vi "RunTest.vi"(8 "error in":errorcluster, 11 "Prueba31 in":refnum<class "Prueba33.lvclass">) -> (0 "error out":errorcluster, 2 "Resultado":string, 3 "Prueba31 out":refnum<class "Prueba33.lvclass">)   [LabVIEW 2019, in "Prueba33.lvclass"]
uses:
  Prueba33.lvclass
  Prueba04/Control/Slide.ctl
  Controles/Tab.ctl
  <vilib>/Utility/miscctls.llb/LVRowAndColumnTypeDef.ctl
  Prueba33.lvclass/Prueba33.ctl
  QMH/Message Queue/Enqueue Message (Single).vi
  <vilib>/Utility/error.llb/Error Cluster From Error Code.vi
  <vilib>/ErrorRing/Error Ring.xnode
  QMH/Message Queue/Message Queue.lvlib
  QMH/User Event - Stop/User Event - Stop.lvlib
  Prueba04/Prueba04.lvclass
panel:
  in  "Tab":T1
  out "Estatus_MainD4":string
  in  "Configurar_MainD4":bool
  in  "Ver_MainD4":bool
  out "Estatus_MainD3":string
  in  "Configurar_MainD3":bool
  in  "Ver_MainD3":bool
  out "Estatus_MainD2":string
  in  "Configurar_MainD2":bool
  in  "Ver_MainD2":bool
  out "Estatus_MainD1":string
  in  "Configurar_MainD1":bool
  in  "Ver_MainD1":bool
  in  "Salir_Main":bool
  in  "frecuencia_D1A":string(combo)="63"
  out "NivelendB_D1A":dbl=95.0
  out "rangoRef_D1A":string
  in  "guardarVref_D1A":bool
  in  "generar_D1A":bool
  in  "AjusteAmp_D1A":T2 caption="Ajuste de amplitud [mV]" scale=0.0..5000.0
  out "voltajeM_D1A":dbl format="%#.1f"
  out "frecuenciaM_D1A":dbl format="%#.1f"
  in  "seguir_D1A":bool
  in  "Terminar_D1B":bool
  out "Voltaje_D1B":dbl
  in  "generar_D1B":bool
  out "voltajeM_D1B":dbl format="%#.1f"
  out "frecuenciaM_D1B":dbl format="%#.1f"
  in  "salir_D1B":bool
  in  "Tabla_D1B":string[][](table)=[["63"], ["125"], ["250"], ["500"], ["1000"], ["2000"], ["4000"], ["8000"]]
  in  "frecuencia_D1B":string(combo)="63"
  in  "frecuencia_D2A":string(combo)="63"
  in  "seguir_D2A":bool
  out "voltajeM_D2A":dbl format="%#.1f"
  out "frecuenciaM_D2A":dbl format="%#.1f"
  in  "AjusteAmp_D2A":T2 caption="Ajuste de amplitud [mV]" scale=0.0..5000.0
  in  "generar_D2A":bool
  in  "guardarVref_D2A":bool
  out "rangoRef_D2A":string
  out "NivelendB_D2A":dbl=95.0
  in  "Terminar_D2B":bool
  in  "frecuencia_D2B":string(combo)="63"
  in  "salir_D2B":bool
  out "voltajeM_D2B":dbl format="%#.1f"
  out "frecuenciaM_D2B":dbl format="%#.1f"
  in  "generar_D2B":bool
  out "Voltaje_D2B":dbl
  in  "Tabla_D2B":string[][](table)=[["63"], ["125"], ["250"], ["500"], ["1000"], ["2000"], ["4000"], ["8000"]]
  in  "frecuencia_D3A":string(combo)="63"
  out "NivelendB_D3A":dbl=95.0
  out "rangoRef_D3A":string
  in  "guardarVref_D3A":bool
  in  "generar_D3A":bool
  in  "AjusteAmp_D3A":T2 caption="Ajuste de amplitud [mV]" scale=0.0..5000.0
  out "voltajeM_D3A":dbl format="%#.1f"
  out "frecuenciaM_D3A":dbl format="%#.1f"
  in  "seguir_D3A":bool
  in  "Terminar_D3B":bool
  in  "frecuencia_D3B":string(combo)="63"
  in  "Tabla_D3B":string[][](table)=[["63"], ["125"], ["250"], ["500"], ["1000"], ["2000"], ["4000"], ["8000"]]
  out "Voltaje_D3B":dbl
  in  "generar_D3B":bool
  out "voltajeM_D3B":dbl format="%#.1f"
  out "frecuenciaM_D3B":dbl format="%#.1f"
  in  "salir_D3B":bool
  in  "frecuencia_D4A":string(combo)="63"
  in  "seguir_D4A":bool
  out "voltajeM_D4A":dbl format="%#.1f"
  out "frecuenciaM_D4A":dbl format="%#.1f"
  in  "AjusteAmp_D4A":T2 caption="Ajuste de amplitud [mV]" scale=0.0..5000.0
  in  "generar_D4A":bool
  in  "guardarVref_D4A":bool
  out "rangoRef_D4A":string
  out "NivelendB_D4A":dbl=95.0
  in  "Terminar_D4B":bool
  in  "salir_D4B":bool
  out "voltajeM_D4B":dbl format="%#.1f"
  out "frecuenciaM_D4B":dbl format="%#.1f"
  in  "generar_D4B":bool
  out "Voltaje_D4B":dbl
  in  "Tabla_D4B":string[][](table)=[["63"], ["125"], ["250"], ["500"], ["1000"], ["2000"], ["4000"], ["8000"]]
  in  "frecuencia_D4B":string(combo)="63"
  # "Vienen de base de datos\nambos\ncambiar a numerico indicador"
  # "Dosimetro 4"
  # "Dosimetro 3"
  # "Dosimetro 2"
  # "Dosimetro 1"
  # "3.  Ponderación frecuencial A (entrada eléctrica). . IEC 61252: 2002 Cláusula 7"
  # "Elección Señal de Referencia\nsegún marca y modelo de sonómetro"
  # "Nivel en dB"
  # "Rango Referencia"
  # "Frecuencia"
  # "Monitoreo"
  # "Frecuencia"
  # "Hz"
  # "Voltaje"
  # "mV"
  # "3.  Ponderación frecuencial A (entrada eléctrica). . IEC 61252: 2002 Cláusula 7\nDosimetro 1"
  # "Tabla Resultados"
  # "3.  Ponderación frecuencial A (entrada eléctrica). . IEC 61252: 2002 Cláusula 7\nDosimetro 1"
  # "Voltaje"
  # "Frecuencia"
  # "Monitoreo"
  # "Frecuencia"
  # "Hz"
  # "Voltaje"
  # "mV"
  # "Elección Señal de Referencia\nsegún marca y modelo de sonómetro"
  # "3.  Ponderación frecuencial A (entrada eléctrica). . IEC 61252: 2002 Cláusula 7\nDosimetro 2"
  # "Monitoreo"
  # "Frecuencia"
  # "Hz"
  # "Voltaje"
  # "mV"
  # "Frecuencia"
  # "Rango Referencia"
  # "Nivel en dB"
  # "Tabla Resultados"
  # "3.  Ponderación frecuencial A (entrada eléctrica). . IEC 61252: 2002 Cláusula 7\nDosimetro 2"
  # "Monitoreo"
  # "Frecuencia"
  # "Hz"
  # "Voltaje"
  # "mV"
  # "Frecuencia"
  # "Voltaje"
  # "Elección Señal de Referencia\nsegún marca y modelo de sonómetro"
  # "3.  Ponderación frecuencial A (entrada eléctrica). . IEC 61252: 2002 Cláusula 7\nDosimetro 3"
  # "Nivel en dB"
  # "Rango Referencia"
  # "Frecuencia"
  # "Monitoreo"
  # "Frecuencia"
  # "Hz"
  # "Voltaje"
  # "mV"
  # "Tabla Resultados"
  # "3.  Ponderación frecuencial A (entrada eléctrica). . IEC 61252: 2002 Cláusula 7\nDosimetro 3"
  # "Voltaje"
  # "Frecuencia"
  # "Monitoreo"
  # "Frecuencia"
  # "Hz"
  # "Voltaje"
  # "mV"
  # "Elección Señal de Referencia\nsegún marca y modelo de sonómetro"
  # "3.  Ponderación frecuencial A (entrada eléctrica). . IEC 61252: 2002 Cláusula 7\nDosimetro 4"
  # "Monitoreo"
  # "Frecuencia"
  # "Hz"
  # "Voltaje"
  # "mV"
  # "Frecuencia"
  # "Rango Referencia"
  # "Nivel en dB"
  # "Tabla Resultados"
  # "Monitoreo"
  # "Frecuencia"
  # "Hz"
  # "Voltaje"
  # "mV"
  # "Frecuencia"
  # "Voltaje"
  # "3.  Ponderación frecuencial A (entrada eléctrica). . IEC 61252: 2002 Cláusula 7\nDosimetro 4"
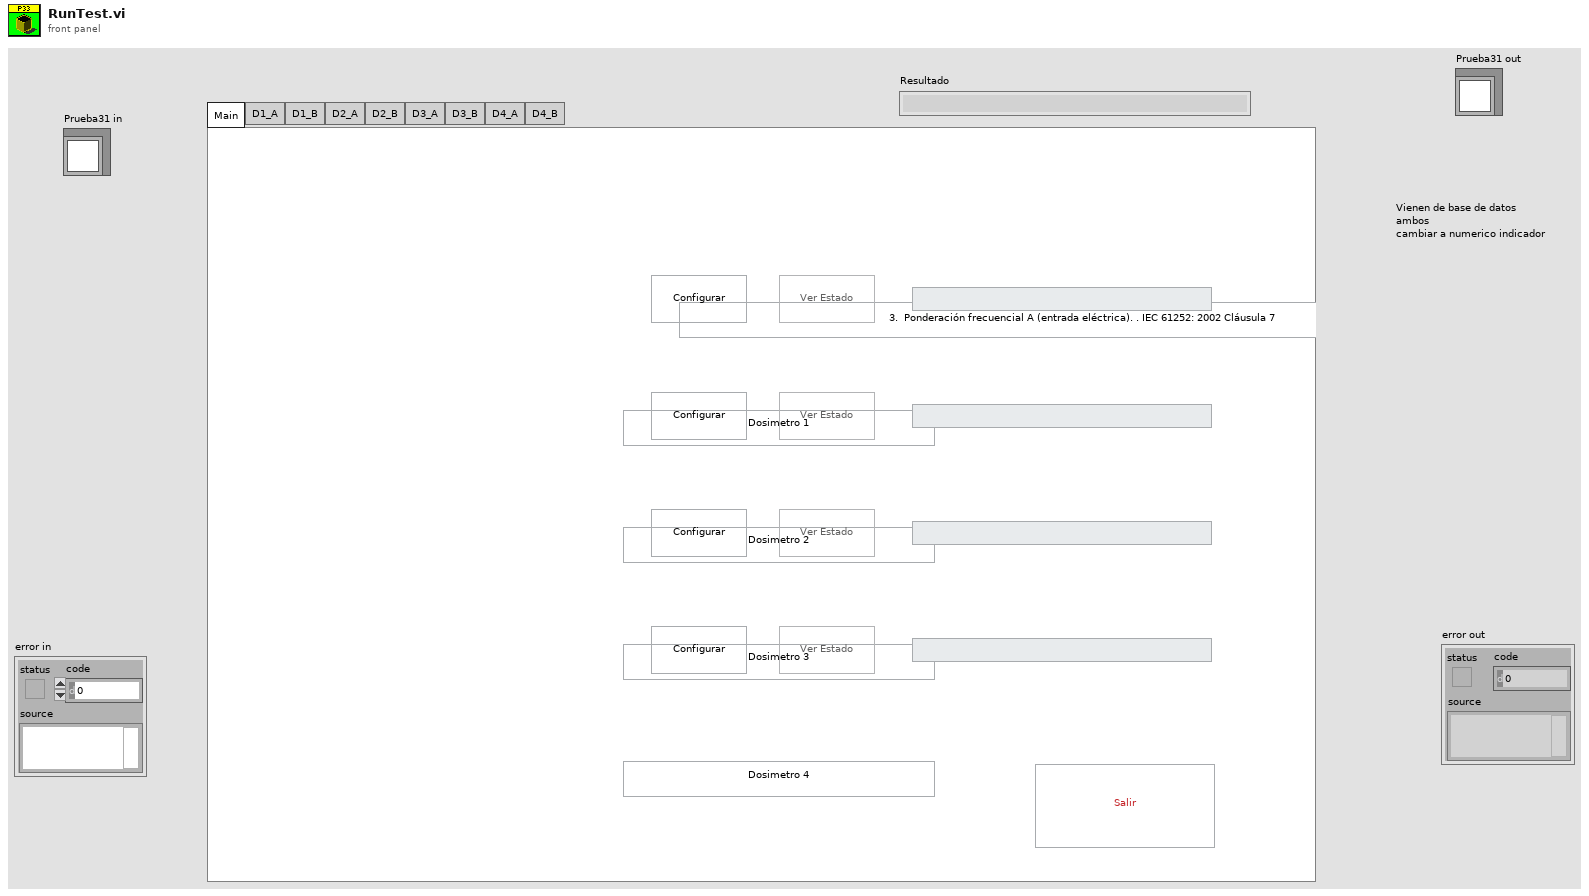
[diagram p1: front panel]
types:
  T1 = typedef "Prueba33.lvclass/Tab.ctl" = enum32{"Main", "D1_A", "D1_B", "D2_A", "D2_B", "D3_A", "D3_B", "D4_A", "D4_B"}
  T2 = typedef "Prueba04.lvclass/Slide.ctl" = dbl
  T3 = typedef "Message Queue.lvlib/All Message Queues.ctl" = cluster{"MHL":refnum<queue>, "Inst_CNT90":refnum<queue>, "Inst_DS360":refnum<queue>, "Inst_Keithley2002":refnum<queue>, "Inst_DAQ":refnum<queue>, "BD":refnum<queue>, "Pistofono":refnum<queue>, "Nexus":refnum<queue>}
  T4 = typedef "LVRowAndColumnTypeDef.ctl" = cluster{"Row":i32, "Column":i32}
  T5 = cluster{"Channel 1":cluster{"amplitude":dbl, "detected fundamental frequency":dbl}, "Channel 2":cluster{"amplitude":dbl, "detected fundamental frequency":dbl}, "Channel 3":cluster{"amplitude":dbl, "detected fundamental frequency":dbl}, "Channel 4":cluster{"amplitude":dbl, "detected fundamental frequency":dbl}}
  T6 = cluster{"Vref":dbl, "Frecuencia":dbl, "Channel":string}
  T7 = cluster{"Vref_D1":dbl, "Vref_D2":dbl, "Vref_D3":dbl, "Vref_D4":dbl}
  T8 = cluster{"ControlName":string, "ControlReference":refnum<vi>}[]
  T9 = enum16{"Tabla_D1", "Tabla_D2", "Tabla_D3", "Tabla_D4"}[]
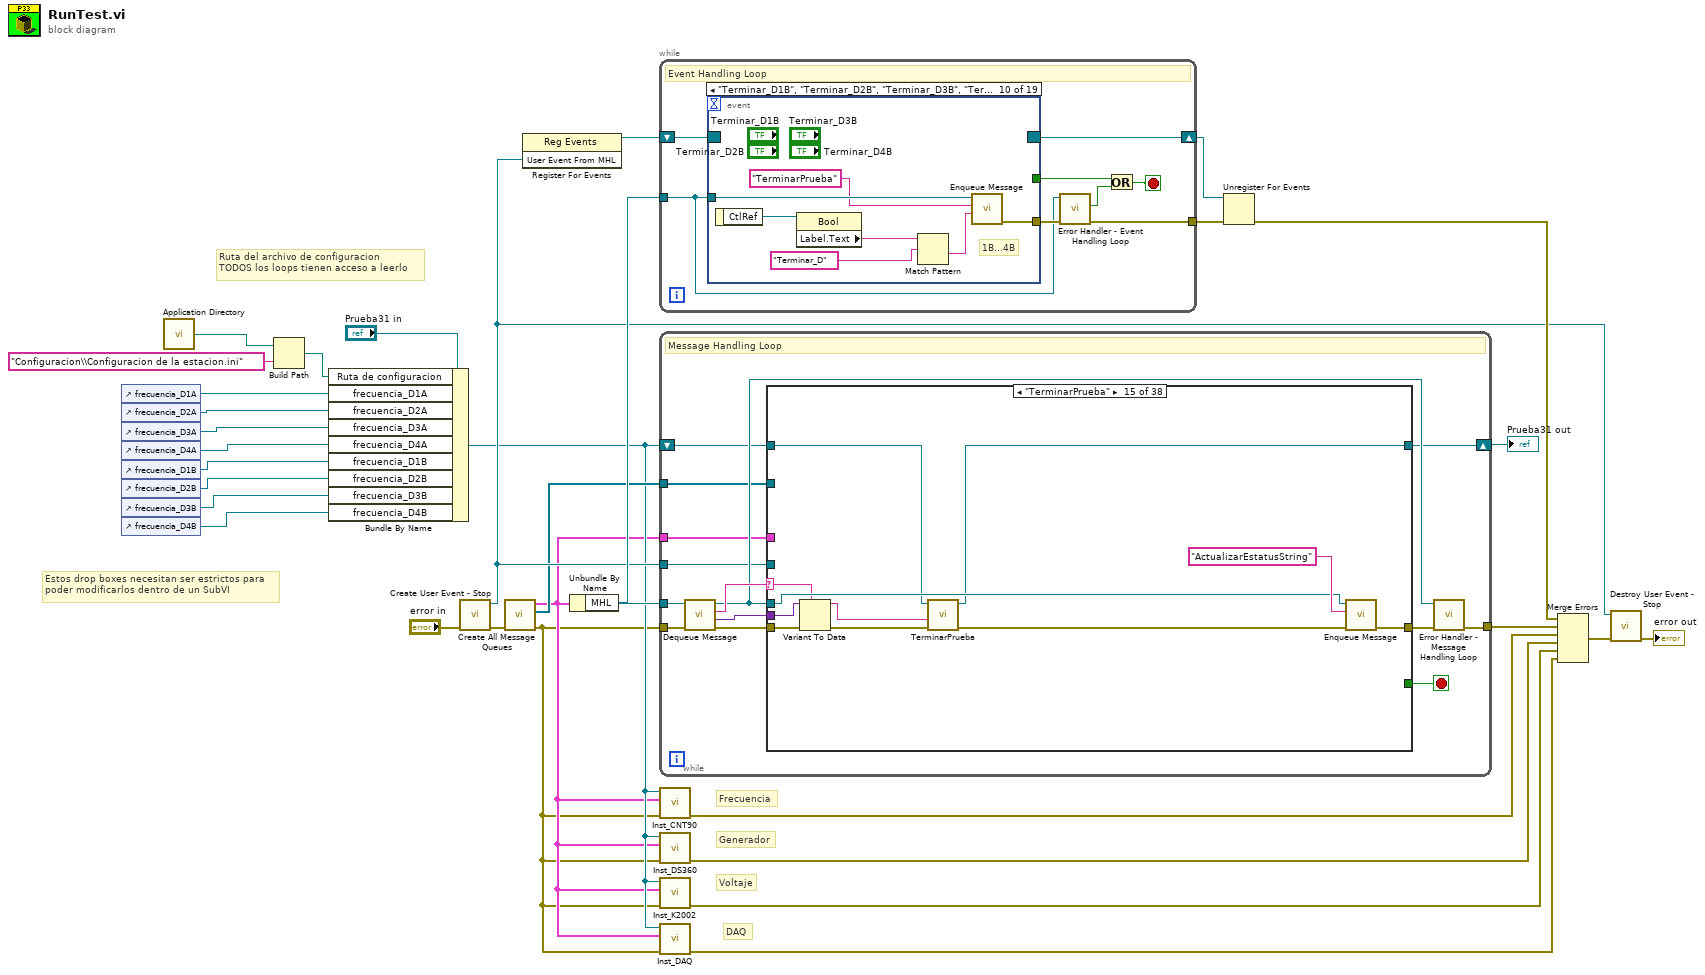
[diagram p0: block diagram]
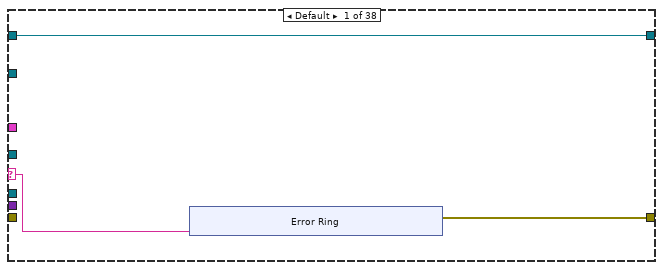
[diagram p2: hidden frame]
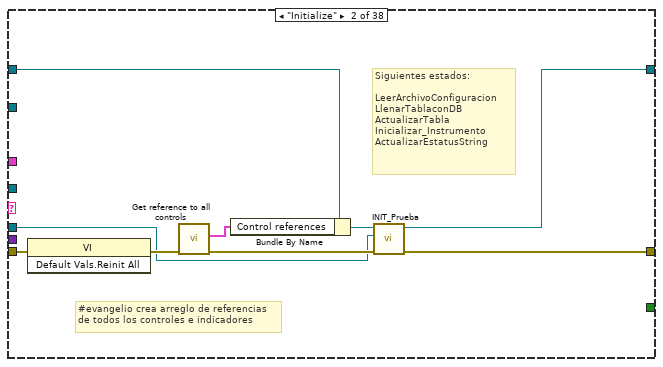
[diagram p3: hidden frame]
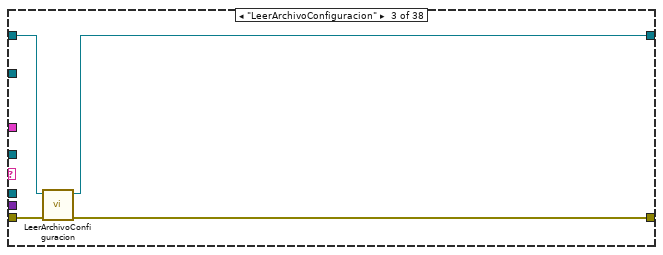
[diagram p4: hidden frame]
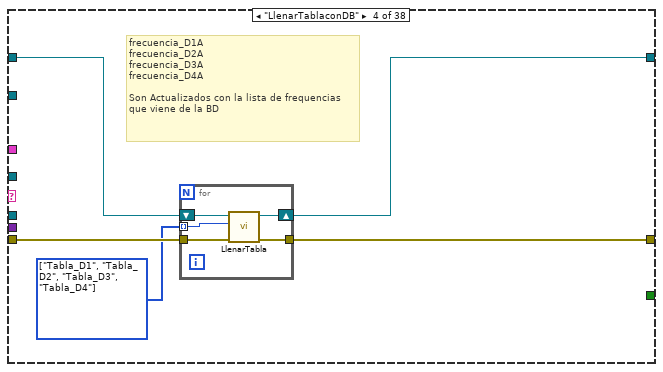
[diagram p5: hidden frame]
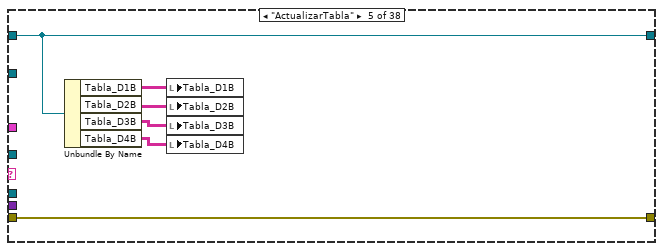
[diagram p6: hidden frame]
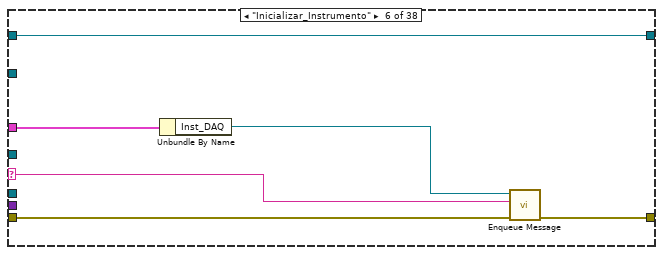
[diagram p7: hidden frame]
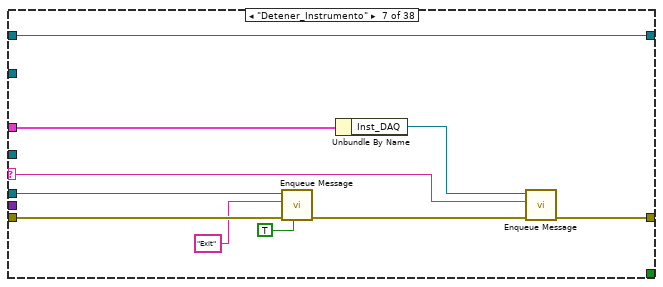
[diagram p8: hidden frame]
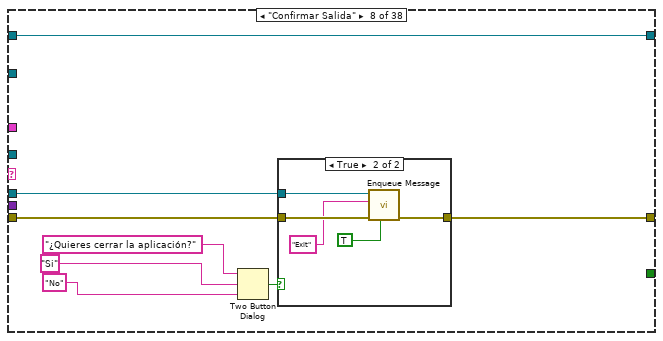
[diagram p9: hidden frame]
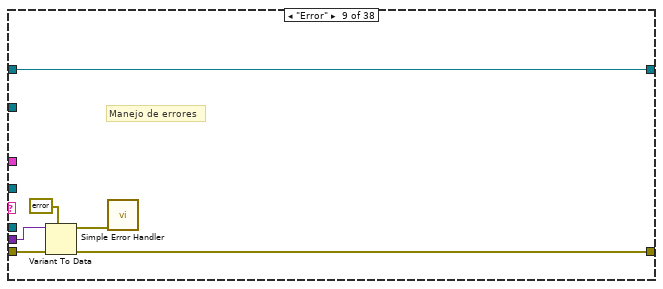
[diagram p11: hidden frame]
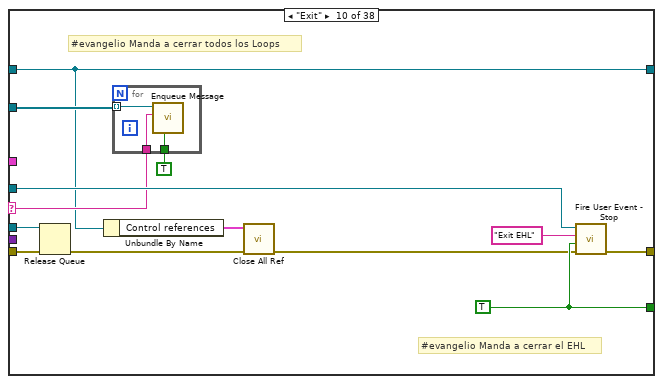
[diagram p12: hidden frame]
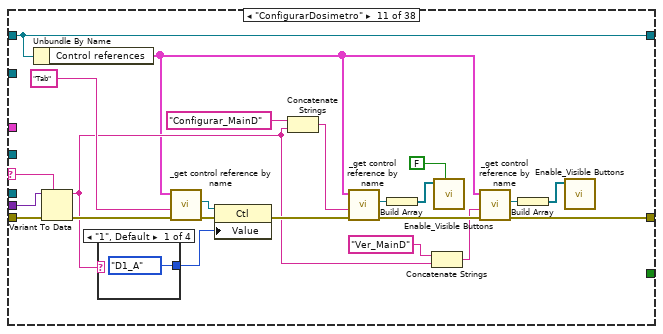
[diagram p13: hidden frame]
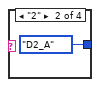
[diagram p14: hidden frame]
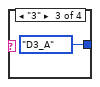
[diagram p15: hidden frame]
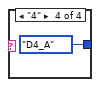
[diagram p16: hidden frame]
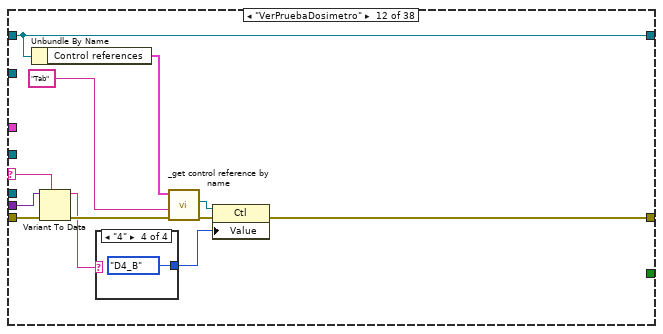
[diagram p17: hidden frame]
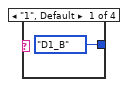
[diagram p18: hidden frame]
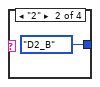
[diagram p19: hidden frame]
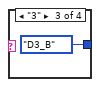
[diagram p20: hidden frame]
diagram:
  # "Ruta del archivo de configuracion\nTODOS los loops tienen acceso a leerlo"
  # "Estos drop boxes necesitan ser estrictos para\npoder modificarlos dentro de un SubVI"
  # "DAQ"
  # "Generador"
  # "Voltaje"
  # "Frecuencia"
  n1 = control-ref of="frecuencia_D1A"() -> (w8:refnum<vi>)
  n2 = control-ref of="frecuencia_D2A"() -> (w7:refnum<vi>)
  n3 = control-ref of="frecuencia_D3A"() -> (w6:refnum<vi>)
  n4 = control-ref of="frecuencia_D4A"() -> (w5:refnum<vi>)
  n5 = control-ref of="frecuencia_D1B"() -> (w4:refnum<vi>)
  n6 = control-ref of="frecuencia_D2B"() -> (w3:refnum<vi>)
  n7 = control-ref of="frecuencia_D3B"() -> (w2:refnum<vi>)
  n8 = control-ref of="frecuencia_D4B"() -> (w1:refnum<vi>)
  n9 = call <vilib>:"Application Directory.vi"() -> ("Application Directory"=w16:path)
  n10 = Build Path(base path=w16, name or relative path="Configuracion\\Configuracion de la estacion.ini") -> (appended path=w15:path)
  n11 = Bundle By Name(cluster="Prueba31 in", "Ruta de configuracion"=w15, "frecuencia_D1A"=w8, "frecuencia_D2A"=w7, "frecuencia_D3A"=w6, "frecuencia_D4A"=w5, "frecuencia_D1B"=w4, "frecuencia_D2B"=w3, "frecuencia_D3B"=w2, "frecuencia_D4B"=w1) -> (w12:refnum<class "Prueba33.lvclass">)
  n12 = call "Create User Event - Stop.vi"("error in (no error)"="error in") -> ("error out"=w29:errorcluster, "User Event From MHL"=w23:refnum<user-event>)  [unwired: 9 in]
  n13 = call "Create All Message Queues.vi"("error in (no error)"=w29) -> ("error out"=w10:errorcluster, "PL Queues Array"=w13:refnum<queue>[], "All Message Queues out"=w11:T3)  [unwired: 8 in]
  n14 = register-events(w23) -> (reference out=w32:refnum<event-registration>)  [unwired: 2 in, 1 out]
  n15 = Unbundle By Name(w11) -> ("MHL"=w28:refnum<queue>)
  n16 = while {
    tunnel: w28 -> [w33]
    tunnel: [w37] -> w31
    shift-right: [w39] -> w30
    shift-left: w32 -> [w40]
    stop <- w34 stop-if-true
    # "Event Handling Loop"
    n17 = event shown="[9] \"Terminar_D1B\", \"Terminar_D2B\", \"Terminar_D3B\", \"Terminar_D4B\": Value Change" {
      selector: w40 -> [_ _ _ _ _ _ _ _ _ _ _ _ _ _ _ _ _ _ _]
      dyn-events: [_ _ _ _ _ _ _ _ _ _ _ _ _ _ _ _ _ _ _] -> w39
      timeout: _ -> [_ _ _ _ _ _ _ _ _ _ _ _ _ _ _ _ _ _ _]
      tunnel: w33 -> [w43 _ w52 w59 w66 w73 w80 w87 w94 w101 w110 w121 w131 w141 w151 w161 w171 w181 w183]
      tunnel: [w44 _ w53 w60 w67 w74 w81 w88 w95 w102 w111 w122 w132 w142 w152 w162 w172 w182 w192] -> w38
      tunnel: [_ w45 _ _ _ _ _ _ _ _ _ _ _ _ _ _ _ _ _] -> w35
      event Panel Close? {
        w41 = TRUE
        n18 = event-data() -> ()  [unwired: 1 in, 1 out]
        n19 = call-poly "Enqueue Message.vi"("Priority Message? (F)"=w41, "Message"="Confirmar Salida", "Message Queue"=w43) -> ("error out"=w44:errorcluster)  [unwired: 7 in, 1 out]
        n20 = event-data("Discard?"=w41) -> ()  [unwired: 1 in, 1 out]
      }
      event User Event {
        n21 = event-data() -> ("User Event"=w47:string, "Event Data"=w46:variant)  [unwired: 1 in]
        n22 = case shown="Default" w47 {
          tunnel: w46 -> [_ w49]
          tunnel: [_ w48] -> w45
          frame Default {
          }
          frame "Exit EHL" {
            # "#evangelio Termina\nla ejecucion del EHL"
            n23 = Variant To Data(type=TRUE, Variant=w49) -> (data=w48:bool)  [unwired: 1 in, 1 out]
          }
        }
      }
      event "Salir_Main": Value Change {
        n24 = event-data() -> ()  [unwired: 1 in, 1 out]
        n25 = call-poly "Enqueue Message.vi"("Message"="Detener_Instrumento", "Message Queue"=w52) -> ("error out"=w53:errorcluster)  [unwired: 8 in, 1 out]
      }
      event "Configurar_MainD1", "Configurar_MainD2", "Configurar_MainD3", "Configurar_MainD4": Value Change {
        n26 = event-data() -> ("CtlRef"=w57:refnum<vi>)  [unwired: 1 in]
        n27 = property class="Bool"(reference=w57) -> ("Label.Text"=w56:string)  [unwired: 1 in, 2 out]
        n28 = Match Pattern(string=w56, regular expression="Configurar_MainD" ("Message")) -> (after substring=w54:string)  [unwired: 1 in, 3 out]
        n29 = call-poly "Enqueue Message.vi"("Message Data"=w54, "Message"="ConfigurarDosimetro", "Message Queue"=w59) -> ("error out"=w60:errorcluster)  [unwired: 7 in, 1 out]
      }
      event "Ver_MainD1", "Ver_MainD2", "Ver_MainD3", "Ver_MainD4": Value Change {
        n30 = event-data() -> ("CtlRef"=w64:refnum<vi>)  [unwired: 1 in]
        n31 = property class="Bool"(reference=w64) -> ("Label.Text"=w63:string)  [unwired: 1 in, 2 out]
        n32 = Match Pattern(string=w63, regular expression="Ver_MainD" ("Message")) -> (after substring=w61:string)  [unwired: 1 in, 3 out]
        n33 = call-poly "Enqueue Message.vi"("Message Data"=w61, "Message"="VerPruebaDosimetro", "Message Queue"=w66) -> ("error out"=w67:errorcluster)  [unwired: 7 in, 1 out]
      }
      event "seguir_D1A", "seguir_D2A", "seguir_D3A", "seguir_D4A": Value Change {
        n34 = event-data() -> ("CtlRef"=w71:refnum<vi>)  [unwired: 1 in]
        n35 = property class="Bool"(reference=w71) -> ("Label.Text"=w70:string)  [unwired: 1 in, 2 out]
        n36 = Match Pattern(string=w70, regular expression="seguir_D" ("Message")) -> (after substring=w68:string)  [unwired: 1 in, 3 out]
        n37 = call-poly "Enqueue Message.vi"("Message Data"=w68, "Message"="MoveraPruebaB", "Message Queue"=w73) -> ("error out"=w74:errorcluster)  [unwired: 7 in, 1 out]
      }
      event "salir_D1B", "salir_D2B", "salir_D3B", "salir_D4B": Value Change {
        n38 = event-data() -> ("CtlRef"=w78:refnum<vi>)  [unwired: 1 in]
        n39 = property class="Bool"(reference=w78) -> ("Label.Text"=w77:string)  [unwired: 1 in, 2 out]
        n40 = Match Pattern(string=w77, regular expression="salir_D" ("Message")) -> (after substring=w75:string)  [unwired: 1 in, 3 out]
        n41 = call-poly "Enqueue Message.vi"("Message Data"=w75, "Message"="MoveraPruebaMain", "Message Queue"=w80) -> ("error out"=w81:errorcluster)  [unwired: 7 in, 1 out]
      }
      event Value Change {
        # "1A...4A"
        n42 = event-data() -> ("CtlRef"=w85:refnum<vi>)  [unwired: 1 in]
        n43 = property class="Slide (strict)"(reference=w85) -> ("Label.Text"=w84:string)  [unwired: 1 in, 2 out]
        n44 = Match Pattern(string=w84, regular expression="AjusteAmp_D" ("Message")) -> (after substring=w82:string)  [unwired: 1 in, 3 out]
        n45 = call-poly "Enqueue Message.vi"("Message Data"=w82, "Message"="AjustarAmplitud", "Message Queue"=w87) -> ("error out"=w88:errorcluster)  [unwired: 7 in, 1 out]
      }
      event "guardarVref_D1A", "guardarVref_D2A", "guardarVref_D3A", "guardarVref_D4A": Value Change {
        # "1A...4A"
        n46 = event-data() -> ("CtlRef"=w92:refnum<vi>)  [unwired: 1 in]
        n47 = property class="Bool"(reference=w92) -> ("Label.Text"=w91:string)  [unwired: 1 in, 2 out]
        n48 = Match Pattern(string=w91, regular expression="guardarVref_D" ("Message")) -> (after substring=w89:string)  [unwired: 1 in, 3 out]
        n49 = call-poly "Enqueue Message.vi"("Message Data"=w89, "Message"="GuardarVref", "Message Queue"=w94) -> ("error out"=w95:errorcluster)  [unwired: 7 in, 1 out]
      }
      event "Terminar_D1B", "Terminar_D2B", "Terminar_D3B", "Terminar_D4B": Value Change {
        # "1B...4B"
        n50 = event-data() -> ("CtlRef"=w99:refnum<vi>)  [unwired: 1 in]
        n51 = property class="Bool"(reference=w99) -> ("Label.Text"=w98:string)  [unwired: 1 in, 2 out]
        n52 = Match Pattern(string=w98, regular expression="Terminar_D" ("Message")) -> (after substring=w96:string)  [unwired: 1 in, 3 out]
        n53 = call-poly "Enqueue Message.vi"("Message Data"=w96, "Message"="TerminarPrueba", "Message Queue"=w101) -> ("error out"=w102:errorcluster)  [unwired: 7 in, 1 out]
      }
      event "generar_D1A": Value Change {
        # "1A...4A"
        n54 = event-data() -> ("CtlRef"=w104:refnum<vi>)  [unwired: 1 in]
        n55 = property class="Bool (strict)"(reference=w104) -> ("Label.Text"=w106:string)  [unwired: 1 in, 2 out]
        n56 = Select(t="SetDAQ_AO", s="generar_D1A", f="DetenerMonitor") -> (s? t:f=w107:string)
        n57 = Match Pattern(string=w106, regular expression="generar_D" ("Message")) -> (after substring=w103:string)  [unwired: 1 in, 3 out]
        n58 = call-poly "Enqueue Message.vi"("Message Data"=w103, "Message"=w107, "Message Queue"=w110) -> ("error out"=w111:errorcluster)  [unwired: 7 in, 1 out]
      }
      event "generar_D2A": Value Change {
        # "1A...4A"
        n59 = event-data() -> ("CtlRef"=w115:refnum<vi>)  [unwired: 1 in]
        n60 = property class="Bool (strict)"(reference=w115) -> ("Label.Text"=w117:string)  [unwired: 1 in, 2 out]
        n61 = Select(t="SetDAQ_AO", s="generar_D2A", f="DetenerMonitor") -> (s? t:f=w118:string)
        n62 = Match Pattern(string=w117, regular expression="generar_D" ("Message")) -> (after substring=w114:string)  [unwired: 1 in, 3 out]
        n63 = call-poly "Enqueue Message.vi"("Message Data"=w114, "Message"=w118, "Message Queue"=w121) -> ("error out"=w122:errorcluster)  [unwired: 7 in, 1 out]
      }
      event "generar_D3A": Value Change {
        # "1A...4A"
        n64 = event-data() -> ("CtlRef"=w125:refnum<vi>)  [unwired: 1 in]
        n65 = property class="Bool (strict)"(reference=w125) -> ("Label.Text"=w127:string)  [unwired: 1 in, 2 out]
        n66 = Select(t="SetDAQ_AO", s="generar_D3A", f="DetenerMonitor") -> (s? t:f=w128:string)
        n67 = Match Pattern(string=w127, regular expression="generar_D" ("Message")) -> (after substring=w124:string)  [unwired: 1 in, 3 out]
        n68 = call-poly "Enqueue Message.vi"("Message Data"=w124, "Message"=w128, "Message Queue"=w131) -> ("error out"=w132:errorcluster)  [unwired: 7 in, 1 out]
      }
      event "generar_D4A": Value Change {
        # "1A...4A"
        n69 = event-data() -> ("CtlRef"=w135:refnum<vi>)  [unwired: 1 in]
        n70 = property class="Bool (strict)"(reference=w135) -> ("Label.Text"=w137:string)  [unwired: 1 in, 2 out]
        n71 = Select(t="SetDAQ_AO", s="generar_D4A", f="DetenerMonitor") -> (s? t:f=w138:string)
        n72 = Match Pattern(string=w137, regular expression="generar_D" ("Message")) -> (after substring=w134:string)  [unwired: 1 in, 3 out]
        n73 = call-poly "Enqueue Message.vi"("Message Data"=w134, "Message"=w138, "Message Queue"=w141) -> ("error out"=w142:errorcluster)  [unwired: 7 in, 1 out]
      }
      event "generar_D1B": Value Change {
        # "1B...4B"
        n74 = event-data() -> ("CtlRef"=w145:refnum<vi>)  [unwired: 1 in]
        n75 = property class="Bool (strict)"(reference=w145) -> ("Label.Text"=w147:string)  [unwired: 1 in, 2 out]
        n76 = Select(t="SetDAQ_AO", s="generar_D1B", f="DetenerMonitor") -> (s? t:f=w148:string)
        n77 = Match Pattern(string=w147, regular expression="generar_D" ("Message")) -> (after substring=w144:string)  [unwired: 1 in, 3 out]
        n78 = call-poly "Enqueue Message.vi"("Message Data"=w144, "Message"=w148, "Message Queue"=w151) -> ("error out"=w152:errorcluster)  [unwired: 7 in, 1 out]
      }
      event "generar_D2B": Value Change {
        # "1B...4B"
        n79 = event-data() -> ("CtlRef"=w155:refnum<vi>)  [unwired: 1 in]
        n80 = property class="Bool (strict)"(reference=w155) -> ("Label.Text"=w157:string)  [unwired: 1 in, 2 out]
        n81 = Select(t="SetDAQ_AO", s="generar_D2B", f="DetenerMonitor") -> (s? t:f=w158:string)
        n82 = Match Pattern(string=w157, regular expression="generar_D" ("Message")) -> (after substring=w154:string)  [unwired: 1 in, 3 out]
        n83 = call-poly "Enqueue Message.vi"("Message Data"=w154, "Message"=w158, "Message Queue"=w161) -> ("error out"=w162:errorcluster)  [unwired: 7 in, 1 out]
      }
      event "generar_D3B": Value Change {
        # "1B...4B"
        n84 = event-data() -> ("CtlRef"=w165:refnum<vi>)  [unwired: 1 in]
        n85 = property class="Bool (strict)"(reference=w165) -> ("Label.Text"=w167:string)  [unwired: 1 in, 2 out]
        n86 = Select(t="SetDAQ_AO", s="generar_D3B", f="DetenerMonitor") -> (s? t:f=w168:string)
        n87 = Match Pattern(string=w167, regular expression="generar_D" ("Message")) -> (after substring=w164:string)  [unwired: 1 in, 3 out]
        n88 = call-poly "Enqueue Message.vi"("Message Data"=w164, "Message"=w168, "Message Queue"=w171) -> ("error out"=w172:errorcluster)  [unwired: 7 in, 1 out]
      }
      event "generar_D4B": Value Change {
        # "1B...4B"
        n89 = event-data() -> ("CtlRef"=w175:refnum<vi>)  [unwired: 1 in]
        n90 = property class="Bool (strict)"(reference=w175) -> ("Label.Text"=w177:string)  [unwired: 1 in, 2 out]
        n91 = Select(t="SetDAQ_AO", s="generar_D4B", f="DetenerMonitor") -> (s? t:f=w178:string)
        n92 = Match Pattern(string=w177, regular expression="generar_D" ("Message")) -> (after substring=w174:string)  [unwired: 1 in, 3 out]
        n93 = call-poly "Enqueue Message.vi"("Message Data"=w174, "Message"=w178, "Message Queue"=w181) -> ("error out"=w182:errorcluster)  [unwired: 7 in, 1 out]
      }
      event "Tabla_D1B", "Tabla_D2B", "Tabla_D3B", "Tabla_D4B": Value Change {
        # "1B...4B"
        n94 = event-data() -> ("CtlRef"=w191:refnum<vi>)  [unwired: 1 in]
        n95 = property class="Tbl (strict)"(reference=w191) -> ("Selection Start"=w186:T4, "Label.Text"=w188:string)  [unwired: 1 in, 2 out]
        n96 = Match Pattern(string=w188, regular expression="Tabla_D" ("Message")) -> (after substring=w185:string)  [unwired: 1 in, 3 out]
        n97 = Bundle By Name(cluster=cluster{"Tabla":string, "Posicion":T4} {"Tabla"="", "Posicion"={"Row"=0, "Column"=0}}, "Posicion"=w186, "Tabla"=w185) -> (w184:cluster{"Tabla":string, "Posicion":T4})
        n98 = call-poly "Enqueue Message.vi"("Message Data"=w184, "Message"="EvaluarTabla", "Message Queue"=w183) -> ("error out"=w192:errorcluster)  [unwired: 7 in, 1 out]
      }
    }
    n99 = call "Error Handler - Event Handling Loop.vi"("error in (no error)"=w38, "Message Queue"=w33) -> ("dup error in"=w37:errorcluster, "Error?"=w36:bool)  [unwired: 7 in, 1 out]
    n100 = Or(x=w35, y=w36) -> (x .or. y?=w34:bool)
  }
  n101 = while {
    tunnel: w10 -> [w206]
    tunnel: w28 -> [w205]
    tunnel: [w199] -> w26
    shift-right: [w197] -> w24
    shift-left: w12 -> [w198]
    tunnel: w11 -> [w195]
    tunnel: w23 -> [w194]
    tunnel: w13 -> [w193]
    stop <- w196 stop-if-true
    # "Message Handling Loop"
    n102 = call "Dequeue Message.vi"("error in (no error)"=w206, "Message Queue"=w205) -> ("error out"=w202:errorcluster, "Message Data"=w203:variant, "Message"=w204:string, "dup Message Queue"=w201:refnum<queue>)  [unwired: 6 in]
    n103 = case shown="\"TerminarPrueba\"" w204 {
      selector: w204 -> [w208 _ _ _ _ w246 w257 _ _ w286 w318 w326 w346 w371 w394 _ _ _ _ _ _ _ w452 w486 w512 w546 _ _ _ _ _ _ _ _ _ _ _ _]
      tunnel: w201 -> [_ w218 _ _ _ _ w254 w262 _ w293 _ _ _ w367 w397 _ _ _ _ _ _ _ _ _ _ _ _ _ _ _ _ _ _ _ _ _ _ _]
      tunnel: w203 -> [_ _ _ _ _ _ _ _ w277 _ w319 w327 w347 w372 w393 _ _ w420 _ _ _ w442 w460 w489 w517 w550 w560 _ _ _ _ _ _ _ _ _ _ _]
      tunnel: w202 -> [_ w225 w229 w234 w245 w249 w255 w268 w278 w292 w320 w328 w348 w373 w395 w407 w413 w421 w423 w427 w433 w443 w459 w490 w518 w551 w561 w564 w566 w568 w570 w572 w574 w576 w578 w580 w582 w584]
      tunnel: [w207 w217 w226 w231 w245 w250 w260 w267 w279 w290 w300 w325 w344 w368 w398 w407 w413 w417 w423 w428 w434 w439 w455 w494 w513 w547 w562 w564 w566 w568 w570 w572 w574 w576 w578 w580 w582 w584] -> w200
      tunnel: w198 -> [w209 w223 w228 w233 w244 w251 w261 w269 w281 w283 w317 w329 w349 w364 w392 w405 w412 w416 w422 w429 w435 w436 w451 w485 w508 w539 w556 w563 w565 w567 w569 w571 w573 w575 w577 w579 w581 w583]
      tunnel: [w209 w220 w227 w232 w244 w251 w261 w269 w281 w283 w317 w329 w349 w365 w391 w406 w412 w415 w422 w429 w435 w437 w450 w485 w508 w539 w557 w563 w565 w567 w569 w571 w573 w575 w577 w579 w581 w583] -> w197
      tunnel: [_ _ _ _ _ _ _ _ _ w287 _ _ _ _ _ _ _ _ _ _ _ _ _ _ _ _ _ _ _ _ _ _ _ _ _ _ _ _] -> w196
      tunnel: w195 -> [_ _ _ _ _ w248 w259 _ _ _ _ _ w342 _ _ _ _ _ _ w426 w432 _ w454 w493 w510 w544 _ _ _ _ _ _ _ _ _ _ _ _]
      tunnel: w194 -> [_ _ _ _ _ _ _ _ _ w289 _ _ _ _ _ _ _ _ _ _ _ _ _ _ _ _ _ _ _ _ _ _ _ _ _ _ _ _]
      tunnel: w193 -> [_ _ _ _ _ _ _ _ _ w284 _ _ _ _ _ _ _ _ _ _ _ _ _ _ _ _ _ _ _ _ _ _ _ _ _ _ _ _]
      frame Default {
        n104 = xnode "Error Ring"("parameter 0"=w208) -> ("error out"=w207:errorcluster)
      }
      frame "Initialize" {
        # "Siguientes estados:\n\nLeerArchivoConfiguracion\nLlenarTablaconDB\nActualizarTabla\nInicializar_Instrumento\nActualizarEstatusString"
        # "#evangelio crea arreglo de referencias\nde todos los controles e indicadores"
        n105 = invoke class="VI" method="Default Vals.Reinit All"(error in=w225) -> (error out=w224:errorcluster)  [unwired: 2 in, 2 out]
        n106 = call "Get reference to all controls.vi"("error in (no error)"=w224) -> ("error out"=w219:errorcluster, "Control references"=w222:T8)  [unwired: 5 in]
        n107 = Bundle By Name(cluster=w223, "Control references"=w222) -> (w221:refnum<class "Prueba33.lvclass">)
        n108 = call "INIT_Prueba.vi"("error in (no error)"=w219, "dup Message Queue"=w218, "Prueba33 in"=w221) -> ("error out"=w217:errorcluster, "Prueba33 out"=w220:refnum<class "Prueba33.lvclass">)  [unwired: 7 in]
      }
      frame "LeerArchivoConfiguracion" {
        n109 = call "LeerArchivoConfiguracion.vi"("error in"=w229, "Prueba31 in"=w228) -> ("error out"=w226:errorcluster, "Prueba31 out"=w227:refnum<class "Prueba33.lvclass">)  [unwired: 8 in]
      }
      frame "LlenarTablaconDB" {
        w230 = T9 [enum."Tabla_D1", enum."Tabla_D2", enum."Tabla_D3", enum."Tabla_D4"] items=["Tabla_D1", "Tabla_D2", "Tabla_D3", "Tabla_D4"]
        # "frecuencia_D1A\nfrecuencia_D2A\nfrecuencia_D3A\nfrecuencia_D4A\n\nSon Actualizados con la lista de frequencias\nque viene de la BD"
        n110 = for {
          shift-right: [w237] -> w232
          shift-left: w233 -> [w238]
          tunnel: w234 -> [w239]
          tunnel: [w236] -> w231
          tunnel: w230 -> [w235] mode=indexing
          n111 = call "LlenarTabla.vi"("error in (no error)"=w239, "Tabla"=w235, "Prueba32 in"=w238) -> ("error out"=w236:errorcluster, "Prueba32 out"=w237:refnum<class "Prueba33.lvclass">)  [unwired: 7 in]
        }
      }
      frame "ActualizarTabla" {
        n112 = Unbundle By Name(w244) -> ("Tabla_D1B"=w243:string[][], "Tabla_D2B"=w242:string[][], "Tabla_D3B"=w241:string[][], "Tabla_D4B"=w240:string[][])
        n113 = local write "Tabla_D1B"(w243) -> ()
        n114 = local write "Tabla_D2B"(w242) -> ()
        n115 = local write "Tabla_D3B"(w241) -> ()
        n116 = local write "Tabla_D4B"(w240) -> ()
      }
      frame "Inicializar_Instrumento" {
        n117 = Unbundle By Name(w248) -> ("Inst_DAQ"=w247:refnum<queue>)
        n118 = call-poly "Enqueue Message.vi"("error in (no error)"=w249, "Message"=w246, "Message Queue"=w247) -> ("error out"=w250:errorcluster)  [unwired: 7 in, 1 out]
      }
      frame "Detener_Instrumento" {
        n119 = call-poly "Enqueue Message.vi"("Priority Message? (F)"=TRUE, "error in (no error)"=w255, "Message"="Exit", "Message Queue"=w254) -> ("error out"=w256:errorcluster)  [unwired: 6 in, 1 out]
        n120 = Unbundle By Name(w259) -> ("Inst_DAQ"=w258:refnum<queue>)
        n121 = call-poly "Enqueue Message.vi"("error in (no error)"=w256, "Message"=w257, "Message Queue"=w258) -> ("error out"=w260:errorcluster)  [unwired: 7 in, 1 out]
      }
      frame "Confirmar Salida" {
        n122 = Two Button Dialog(message="¿Quieres cerrar la aplicación?", 1:"No" ("T button name (\"OK\")"), 2:"Si" ("T button name (\"OK\")")) -> (T button?=w263:bool)
        n123 = case shown="True" w263 {
          tunnel: w268 -> [w270 w275]
          tunnel: [w270 w274] -> w267
          tunnel: w262 -> [_ w273]
          frame False {
          }
          frame True {
            n124 = call-poly "Enqueue Message.vi"("Priority Message? (F)"=TRUE, "error in (no error)"=w275, "Message"="Exit", "Message Queue"=w273) -> ("error out"=w274:errorcluster)  [unwired: 6 in, 1 out]
          }
        }
      }
      frame "Error" {
        # "Manejo de errores"
        n125 = Variant To Data(error in=w278, type=errorcluster {"status"=FALSE, "code"=0, "source"=""} ("error constant"), Variant=w277) -> (data=w276:errorcluster, error out=w279:errorcluster)
        n126 = call <vilib>:"Simple Error Handler.vi"("error in (no error)"=w276) -> ()  [unwired: 4 in, 5 out]
      }
      frame "Exit" {
        w287 = TRUE
        # "#evangelio Manda a cerrar el EHL"
        # "#evangelio Manda a cerrar todos los Loops"
        n127 = Release Queue(queue=w293, error in (no error)=w292) -> (error out=w291:errorcluster)  [unwired: 1 in, 2 out]
        n128 = Unbundle By Name(w283) -> ("Control references"=w294:T8)
        n129 = for {
          tunnel: w284 -> [w297] mode=indexing
          tunnel: w286 -> [w296]
          tunnel: TRUE -> [w295]
          n130 = call-poly "Enqueue Message.vi"("Priority Message? (F)"=w295, "Message"=w296, "Message Queue"=w297) -> ()  [unwired: 7 in, 2 out]
        }
        n131 = call "Close All Ref.vi"("error in (no error)"=w291, "Control references"=w294) -> ("error out"=w282:errorcluster)  [unwired: 9 in]
        n132 = call "Fire User Event - Stop.vi"("error in (no error)"=w282, "Event Data"=w287, "User Event"="Exit EHL", "User Event in"=w289) -> ("error out"=w290:errorcluster)  [unwired: 7 in]
      }
      frame "ConfigurarDosimetro" {
        n133 = Unbundle By Name(w317) -> ("Control references"=w299:T8)
        n134 = Variant To Data(error in=w320, type=w318, Variant=w319) -> (data=w304:string, error out=w316:errorcluster)
        n135 = case shown="\"1\", Default" w304 {
          tunnel: [Tab."D1_A" ("Tab") Tab."D2_A" ("Tab") Tab."D3_A" ("Tab") Tab."D4_A" ("Tab")] -> w312
          frame "1", Default {
          }
          frame "2" {
          }
          frame "3" {
          }
          frame "4" {
          }
        }
        n136 = call "_get control reference by name.vi"("error in (no error)"=w316, "Control name"="Tab" ("Message"), "Control references"=w299) -> ("error out"=w313:errorcluster, "Ctl Refnum"=w314:refnum<vi>)  [unwired: 3 in]
        n137 = property class="Ctl"(reference=w314, error in=w313, "Value"=w312) -> (error out=w311:errorcluster)  [unwired: 1 out]
        n138 = Concatenate Strings("Configurar_MainD" ("Message"), w304) -> (w309:string)
        n139 = call "_get control reference by name.vi"("error in (no error)"=w311, "Control name"=w309, "Control references"=w299) -> ("error out"=w301:errorcluster, "Ctl Refnum"=w308:refnum<vi>)  [unwired: 3 in]
        n140 = Build Array(w308) -> (w307:refnum<vi>[])
        n141 = Concatenate Strings("Ver_MainD" ("Message"), w304) -> (w298:string)
        n142 = call "Enable_Visible Buttons.vi"("Enable? (T)"=FALSE, "Controls Ref Array"=w307) -> ()  [unwired: 10 in]
        n143 = call "_get control reference by name.vi"("error in (no error)"=w301, "Control name"=w298, "Control references"=w299) -> ("error out"=w300:errorcluster, "Ctl Refnum"=w302:refnum<vi>)  [unwired: 3 in]
        n144 = Build Array(w302) -> (w303:refnum<vi>[])
        n145 = call "Enable_Visible Buttons.vi"("Controls Ref Array"=w303) -> ()  [unwired: 11 in]
      }
      frame "VerPruebaDosimetro" {
        n146 = Unbundle By Name(w329) -> ("Control references"=w330:T8)
        n147 = Variant To Data(error in=w328, type=w326, Variant=w327) -> (data=w331:string, error out=w336:errorcluster)
        n148 = case shown="\"4\"" w331 {
          tunnel: [Tab."D1_B" ("Tab") Tab."D2_B" ("Tab") Tab."D3_B" ("Tab") Tab."D4_B" ("Tab")] -> w332
          frame "1", Default {
          }
          frame "2" {
          }
          frame "3" {
          }
          frame "4" {
          }
        }
        n149 = call "_get control reference by name.vi"("error in (no error)"=w336, "Control name"="Tab" ("Message"), "Control references"=w330) -> ("error out"=w333:errorcluster, "Ctl Refnum"=w334:refnum<vi>)  [unwired: 3 in]
        n150 = property class="Ctl"(reference=w334, error in=w333, "Value"=w332) -> (error out=w325:errorcluster)  [unwired: 1 out]
      }
      frame "MoveraPruebaB" {
        n151 = Unbundle By Name(w349) -> ("Control references"=w350:T8)
        n152 = Variant To Data(error in=w348, type=w346, Variant=w347) -> (data=w351:string, error out=w356:errorcluster)
        n153 = case shown="\"3A\"" w351 {
          tunnel: [Tab."D1_B" ("Tab") Tab."D2_B" ("Tab") Tab."D3_B" ("Tab") Tab."D4_B" ("Tab")] -> w352
          frame "1A", Default {
          }
          frame "2A" {
          }
          frame "3A" {
          }
          frame "4A" {
          }
        }
        n154 = call "_get control reference by name.vi"("error in (no error)"=w356, "Control name"="Tab" ("Message"), "Control references"=w350) -> ("error out"=w353:errorcluster, "Ctl Refnum"=w354:refnum<vi>)  [unwired: 3 in]
        n155 = property class="Ctl"(reference=w354, error in=w353, "Value"=w352) -> (error out=w345:errorcluster)  [unwired: 1 out]
        n156 = Unbundle By Name(w342) -> ("Inst_DAQ"=w341:refnum<queue>)
        n157 = call-poly "Enqueue Message.vi"("error in (no error)"=w345, "Message"="ObtenerVoltajeRefGuardado", "Message Queue"=w341) -> ("error out"=w344:errorcluster)  [unwired: 7 in, 1 out]
      }
      frame "MoveraPruebaMain" {
        n158 = Unbundle By Name(w364) -> ("Control references"=w362:T8)
        n159 = Variant To Data(error in=w373, type=w371, Variant=w372) -> (data=w363:string, error out=w377:errorcluster)
        n160 = call "_get control reference by name.vi"("error in (no error)"=w377, "Control name"="Tab" ("Message"), "Control references"=w362) -> ("error out"=w374:errorcluster, "Ctl Refnum"=w375:refnum<vi>)  [unwired: 3 in]
        n161 = property class="Ctl"(reference=w375, error in=w374, "Value"=Tab."Main" ("Tab")) -> (error out=w369:errorcluster)  [unwired: 1 out]
        n162 = case shown="\"1B\", Default" w363 {
          tunnel: [w380 w383 w386 w389] -> w365
          tunnel: w364 -> [w379 w382 w385 w388]
          tunnel: "Ejecutando Prueba......." ("Message") -> [w378 w381 w384 w387]
          frame "1B", Default {
            n163 = Bundle By Name(cluster=w379, "EstatusStringMain_D1"=w378) -> (w380:refnum<class "Prueba33.lvclass">)
          }
          frame "2B" {
            n164 = Bundle By Name(cluster=w382, "EstatusStringMain_D2"=w381) -> (w383:refnum<class "Prueba33.lvclass">)
          }
          frame "3B" {
            n165 = Bundle By Name(cluster=w385, "EstatusStringMain_D3"=w384) -> (w386:refnum<class "Prueba33.lvclass">)
          }
          frame "4B" {
            n166 = Bundle By Name(cluster=w388, "EstatusStringMain_D4"=w387) -> (w389:refnum<class "Prueba33.lvclass">)
          }
        }
        n167 = call-poly "Enqueue Message.vi"("error in (no error)"=w369, "Message"="ActualizarEstatusString", "Message Queue"=w367) -> ("error out"=w368:errorcluster)  [unwired: 7 in, 1 out]
      }
      frame "TerminarPrueba" {
        n168 = Variant To Data(error in=w395, type=w394, Variant=w393) -> (data=w390:string, error out=w396:errorcluster)
        n169 = call "TerminarPrueba.vi"("error in (no error)"=w396, "String"=w390, "Prueba33 in"=w392) -> ("error out"=w399:errorcluster, "Prueba33 out"=w391:refnum<class "Prueba33.lvclass">)  [unwired: 7 in]
        n170 = call-poly "Enqueue Message.vi"("error in (no error)"=w399, "Message"="ActualizarEstatusString", "Message Queue"=w397) -> ("error out"=w398:errorcluster)  [unwired: 7 in, 1 out]
      }
      frame "ActualizarTablaDatoUsuario" {
        n171 = Bundle By Name(cluster=w405, "Tabla_D1B"="Tabla_D1B", "Tabla_D2B"="Tabla_D2B", "Tabla_D3B"="Tabla_D3B", "Tabla_D4B"="Tabla_D4B") -> (w406:refnum<class "Prueba33.lvclass">)
      }
      frame "ActualizarEstatusString" {
        n172 = Unbundle By Name(w412) -> ("EstatusStringMain_D1"=→"Estatus_MainD1":string, "EstatusStringMain_D2"=→"Estatus_MainD2":string, "EstatusStringMain_D3"=→"Estatus_MainD3":string, "EstatusStringMain_D4"=→"Estatus_MainD4":string)
      }
      frame "EvaluarTabla" {
        n173 = Variant To Data(error in=w421, type=cluster{"Tabla":string, "Posicion":T4} {"Tabla"="", "Posicion"={"Row"=0, "Column"=0}}, Variant=w420) -> (data=w414:cluster{"Tabla":string, "Posicion":T4}, error out=w418:errorcluster)
        n174 = call "EvaluacionTabla.vi"("error in (no error)"=w418, "Cluster"=w414, "Prueba33 in"=w416) -> ("error out"=w417:errorcluster, "Prueba33 out"=w415:refnum<class "Prueba33.lvclass">)  [unwired: 7 in]
      }
      frame "-------Mandar a DAQ--------" {
      }
      frame "IniciarDAQ" {
        n175 = Unbundle By Name(w426) -> ("Inst_DAQ"=w425:refnum<queue>)
        n176 = call-poly "Enqueue Message.vi"("error in (no error)"=w427, "Message"="Inicializar_Instrumento", "Message Queue"=w425) -> ("error out"=w428:errorcluster)  [unwired: 7 in, 1 out]
      }
      frame "DetenerDAQ" {
        n177 = Unbundle By Name(w432) -> ("Inst_DAQ"=w431:refnum<queue>)
        n178 = call-poly "Enqueue Message.vi"("error in (no error)"=w433, "Message"="Detener_Instrumento", "Message Queue"=w431) -> ("error out"=w434:errorcluster)  [unwired: 7 in, 1 out]
      }
      frame "DatoRecibidoDAQ" {
        n179 = Variant To Data(error in=w443, type=T5 {"Channel 1"={"amplitude"=0.0, "detected fundamental frequency"=0.0}, "Channel 2"={"amplitude"=0.0, "detected fundamental frequency"=0.0}, "Channel 3"={"amplitude"=0.0, "detected fundamental frequency"=0.0}, "Channel 4"={"amplitude"=0.0, "detected fundamental frequency"=0.0}}, Variant=w442) -> (data=w438:T5, error out=w440:errorcluster)
        n180 = call "MonitorVoltaje&Frecuencia.vi"("error in (no error)"=w440, "Cluster"=w438, "Prueba33 in"=w436) -> ("error out"=w439:errorcluster, "Prueba33 out"=w437:refnum<class "Prueba33.lvclass">)  [unwired: 7 in]
      }
      frame "AjustarAmplitud" {
        # "Cambio a mV"
        n181 = Variant To Data(error in=w459, type=w452, Variant=w460) -> (data=w458:string, error out=w457:errorcluster)
        n182 = case shown="\"3A\"" w458 {
          selector: w458 -> [w461 w467 w472 w477]
          tunnel: w457 -> [w465 w470 w475 w480]
          tunnel: [w465 w470 w475 w480] -> w456
          tunnel: w451 -> [w464 w469 w474 w479]
          tunnel: [w463 w468 w473 w478] -> w450
          tunnel: ["AjusteAmp_D1A" "AjusteAmp_D2A" "AjusteAmp_D3A" "AjusteAmp_D4A"] -> w445
          tunnel: [w461 w467 w472 w477] -> w444
          frame "1A", Default {
            n183 = Bundle By Name(cluster=w464, "Vref_D1"="AjusteAmp_D1A") -> (w463:refnum<class "Prueba33.lvclass">)
          }
          frame "2A" {
            n184 = Bundle By Name(cluster=w469, "Vref_D2"="AjusteAmp_D2A") -> (w468:refnum<class "Prueba33.lvclass">)
          }
          frame "3A" {
            n185 = Bundle By Name(cluster=w474, "Vref_D3"="AjusteAmp_D3A") -> (w473:refnum<class "Prueba33.lvclass">)
          }
          frame "4A" {
            n186 = Bundle By Name(cluster=w479, "Vref_D4"="AjusteAmp_D4A") -> (w478:refnum<class "Prueba33.lvclass">)
          }
        }
        n187 = Unbundle By Name(w454) -> ("Inst_DAQ"=w453:refnum<queue>)
        n188 = Divide(x=w445, y=1000.0) -> (x/y=w446:T2)
        n189 = Bundle By Name(cluster=cluster{"Amplitud":dbl, "Channel":string} {"Amplitud"=0.0, "Channel"=""}, "Amplitud"=w446, "Channel"=w444) -> (w448:cluster{"Amplitud":dbl, "Channel":string})
        n190 = call-poly "Enqueue Message.vi"("error in (no error)"=w456, "Message Data"=w448, "Message"=w452, "Message Queue"=w453) -> ("error out"=w455:errorcluster)  [unwired: 6 in, 1 out]
      }
      frame "GuardarVref" {
        n191 = Variant To Data(error in=w490, type=w486, Variant=w489) -> (data=w484:string, error out=w491:errorcluster)
        n192 = case shown="\"4A\"" w484 {
          tunnel: w485 -> [w496 w498 w500 w502]
          tunnel: [w495 w497 w499 w501] -> w482
          frame "1A", Default {
            n193 = Unbundle By Name(w496) -> ("Vref_D1"=w495:dbl)
          }
          frame "2A" {
            n194 = Unbundle By Name(w498) -> ("Vref_D2"=w497:dbl)
          }
          frame "3A" {
            n195 = Unbundle By Name(w500) -> ("Vref_D3"=w499:dbl)
          }
          frame "4A" {
            n196 = Unbundle By Name(w502) -> ("Vref_D4"=w501:dbl)
          }
        }
        n197 = Divide(x=w482, y=1000.0) -> (x/y=w481:dbl)
        n198 = Bundle By Name(cluster=cluster{"Vref":dbl, "Channel":string} {"Vref"=0.0, "Channel"=""}, "Vref"=w481, "Channel"=w484) -> (w487:cluster{"Vref":dbl, "Channel":string})
        n199 = Unbundle By Name(w493) -> ("Inst_DAQ"=w492:refnum<queue>)
        n200 = call-poly "Enqueue Message.vi"("error in (no error)"=w491, "Message Data"=w487, "Message"=w486, "Message Queue"=w492) -> ("error out"=w494:errorcluster)  [unwired: 6 in, 1 out]
      }
      frame "SetDAQ_AO" {
        n201 = Variant To Data(error in=w518, type=w512, Variant=w517) -> (data=w514:string, error out=w507:errorcluster)
        n202 = Unbundle By Name(w508) -> ("Control references"=w505:T8)
        n203 = Unbundle By Name(w510) -> ("Inst_DAQ"=w509:refnum<queue>)
        n204 = call "_get mutiple control reference by name.vi"("error in (no error)"=w507, "Control names"=string[] ["AjusteAmp_D1A", "AjusteAmp_D2A", "AjusteAmp_D3A", "AjusteAmp_D4A", "guardarVref_D1A", "guardarVref_D2A", "guardarVref_D3A", "guardarVref_D4A"], "Control references"=w505) -> ("error out"=w506:errorcluster, "References"=w504:refnum<vi>[])  [unwired: 3 in]
        n205 = case shown="\"1B\"" w514 {
          tunnel: [w520 w522 w524 w526 w528 w530 w532 w534] -> w515
          frame "1A", Default {
            n206 = Fract/Exp String To Number(string="frecuencia_D1A") -> (number=w520:dbl)  [unwired: 3 in, 1 out]
          }
          frame "2A" {
            n207 = Fract/Exp String To Number(string="frecuencia_D2A") -> (number=w522:dbl)  [unwired: 3 in, 1 out]
          }
          frame "3A" {
            n208 = Fract/Exp String To Number(string="frecuencia_D3A") -> (number=w524:dbl)  [unwired: 3 in, 1 out]
          }
          frame "4A" {
            n209 = Fract/Exp String To Number(string="frecuencia_D4A") -> (number=w526:dbl)  [unwired: 3 in, 1 out]
          }
          frame "1B" {
            n210 = Fract/Exp String To Number(string="frecuencia_D1B") -> (number=w528:dbl)  [unwired: 3 in, 1 out]
          }
          frame "2B" {
            n211 = Fract/Exp String To Number(string="frecuencia_D2B") -> (number=w530:dbl)  [unwired: 3 in, 1 out]
          }
          frame "3B" {
            n212 = Fract/Exp String To Number(string="frecuencia_D3B") -> (number=w532:dbl)  [unwired: 3 in, 1 out]
          }
          frame "4B" {
            n213 = Fract/Exp String To Number(string="frecuencia_D4B") -> (number=w534:dbl)  [unwired: 3 in, 1 out]
          }
        }
        n214 = call "Enable_Visible Buttons.vi"("Controls Ref Array"=w504) -> ()  [unwired: 11 in]
        n215 = Bundle By Name(cluster=T6 {"Vref"=0.0, "Frecuencia"=0.0, "Channel"=""}, "Frecuencia"=w515, "Channel"=w514) -> (w511:T6)
        n216 = call-poly "Enqueue Message.vi"("error in (no error)"=w506, "Message Data"=w511, "Message"=w512, "Message Queue"=w509) -> ("error out"=w513:errorcluster)  [unwired: 6 in, 1 out]
      }
      frame "DetenerMonitor" {
        w542 = 0.0 ("Vref")
        n217 = Variant To Data(error in=w551, type=w546, Variant=w550) -> (data=w548:string, error out=w541:errorcluster)
        n218 = Unbundle By Name(w539) -> ("Control references"=w538:T8)
        n219 = call "_get mutiple control reference by name.vi"("error in (no error)"=w541, "Control names"=string[] ["AjusteAmp_D1A", "AjusteAmp_D2A", "AjusteAmp_D3A", "AjusteAmp_D4A", "guardarVref_D1A", "guardarVref_D2A", "guardarVref_D3A", "guardarVref_D4A"], "Control references"=w538) -> ("error out"=w540:errorcluster, "References"=w536:refnum<vi>[])  [unwired: 3 in]
        n220 = call "Enable_Visible Buttons.vi"("Enable? (T)"=FALSE, "Controls Ref Array"=w536) -> ()  [unwired: 10 in]
        n221 = Bundle By Name(cluster=T6 {"Vref"=0.0, "Frecuencia"=0.0, "Channel"=""}, "Vref"=w542, "Frecuencia"=w542, "Channel"=w548) -> (w545:T6)
        n222 = Unbundle By Name(w544) -> ("Inst_DAQ"=w543:refnum<queue>)
        n223 = call-poly "Enqueue Message.vi"("error in (no error)"=w540, "Message Data"=w545, "Message"=w546, "Message Queue"=w543) -> ("error out"=w547:errorcluster)  [unwired: 6 in, 1 out]
      }
      frame "ObtenerVoltajeRefGuardado" {
        n224 = Variant To Data(error in=w561, type=T7 {"Vref_D1"=0.0, "Vref_D2"=0.0, "Vref_D3"=0.0, "Vref_D4"=0.0}, Variant=w560) -> (data=w558:T7, error out=w562:errorcluster)
        n225 = Unbundle By Name(w558) -> ("Vref_D1"=w555:dbl, "Vref_D2"=w554:dbl, "Vref_D3"=w553:dbl, "Vref_D4"=w552:dbl)
        "Voltaje_D1B" <- w555
        "Voltaje_D2B" <- w554
        "Voltaje_D3B" <- w553
        "Voltaje_D4B" <- w552
        n226 = Bundle By Name(cluster=w556, "Vref_D1"=w555, "Vref_D2"=w554, "Vref_D3"=w553, "Vref_D4"=w552) -> (w557:refnum<class "Prueba33.lvclass">)
      }
      frame "-------------------------------" {
      }
      frame "--------------------------Contoles---------------------------" {
      }
      frame "---------- Contoles D1 Main ----------" {
      }
      frame "---------- Contoles D1A ----------" {
      }
      frame "---------- Contoles D1B ----------" {
      }
      frame "---------- Contoles D2A ----------" {
      }
      frame "---------- Contoles D2B ----------" {
      }
      frame "---------- Contoles D3A ----------" {
      }
      frame "---------- Contoles D3B ----------" {
      }
      frame "---------- Contoles D4A ----------" {
      }
      frame "---------- Contoles D4B ----------" {
      }
    }
    n227 = call "Error Handler - Message Handling Loop.vi"("error in (no error)"=w200, "Message Queue"=w201) -> ("dup error in"=w199:errorcluster)  [unwired: 8 in, 1 out]
  }
  "Prueba31 out" <- w24
  n228 = call "Inst_CNT90.vi"("error in"=w10, "All Message Queues in"=w11, "Prueba31 in"=w12) -> ("error out"=w20:errorcluster)  [unwired: 8 in]
  n229 = call "Inst_DS360.vi"("error in"=w10, "All Message Queues in"=w11, "Prueba31 in"=w12) -> ("error out"=w19:errorcluster)  [unwired: 8 in]
  n230 = call "Inst_K2002.vi"("error in"=w10, "All Message Queues in"=w11, "Prueba31 in"=w12) -> ("error out"=w18:errorcluster)  [unwired: 8 in]
  n231 = call "Inst_DAQ.vi"("error in"=w10, "All Message Queues in"=w11, "Prueba31 in"=w12) -> ("error out"=w9:errorcluster)  [unwired: 8 in]
  n232 = Unregister For Events(event registration refnum=w30, error in=w31) -> (error out=w27:errorcluster)
  n233 = Merge Errors(w27, w26, w20, w19, w18, w9) -> (w25:errorcluster)
  n234 = call "Destroy User Event - Stop.vi"("error in (no error)"=w25, "User Event"=w23) -> ("error out"=→"error out":errorcluster)  [unwired: 9 in]
